vi "testUDPReciever - Copy 2.vi"() -> ()   [LabVIEW 2012]
panel:
  out "building array":string[](array[string])
  out "channel":u32
  out "header pre":bool[][](array[boolean])
  out "Found Header":bool
  out "word 0 pre":u8[](array[numeric]) format="%02x"
  out "word 1 pre":u8[](array[numeric]) format="%02x"
  out "word 2 pre":u8[](array[numeric]) format="%02x"
  out "word 3 pre":u8[](array[numeric]) format="%02x"
  out "Raw Data Out":string
  out "error post-check":errorcluster
  out "End Reciever Error":errorcluster
  in  "stop reciever":bool
  out "port":u16
  out "error out post-read":errorcluster
  out "error out pre-read":errorcluster
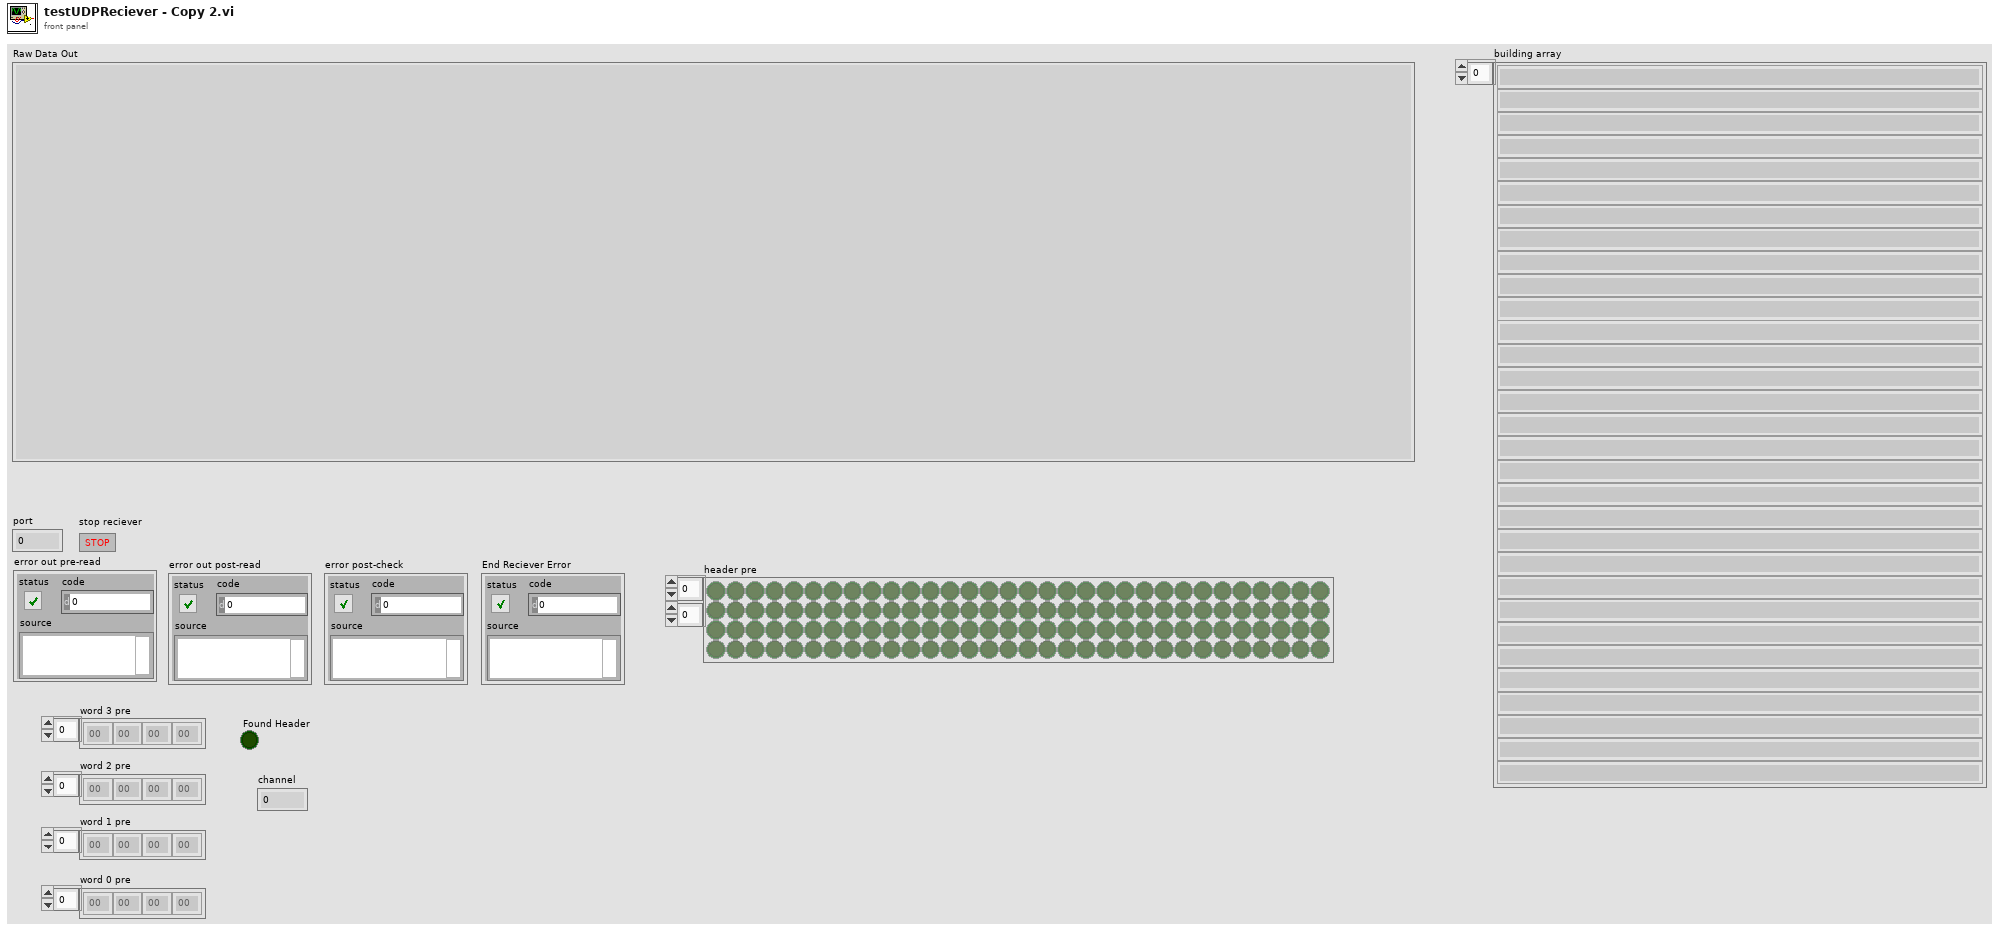
[diagram p1: front panel]
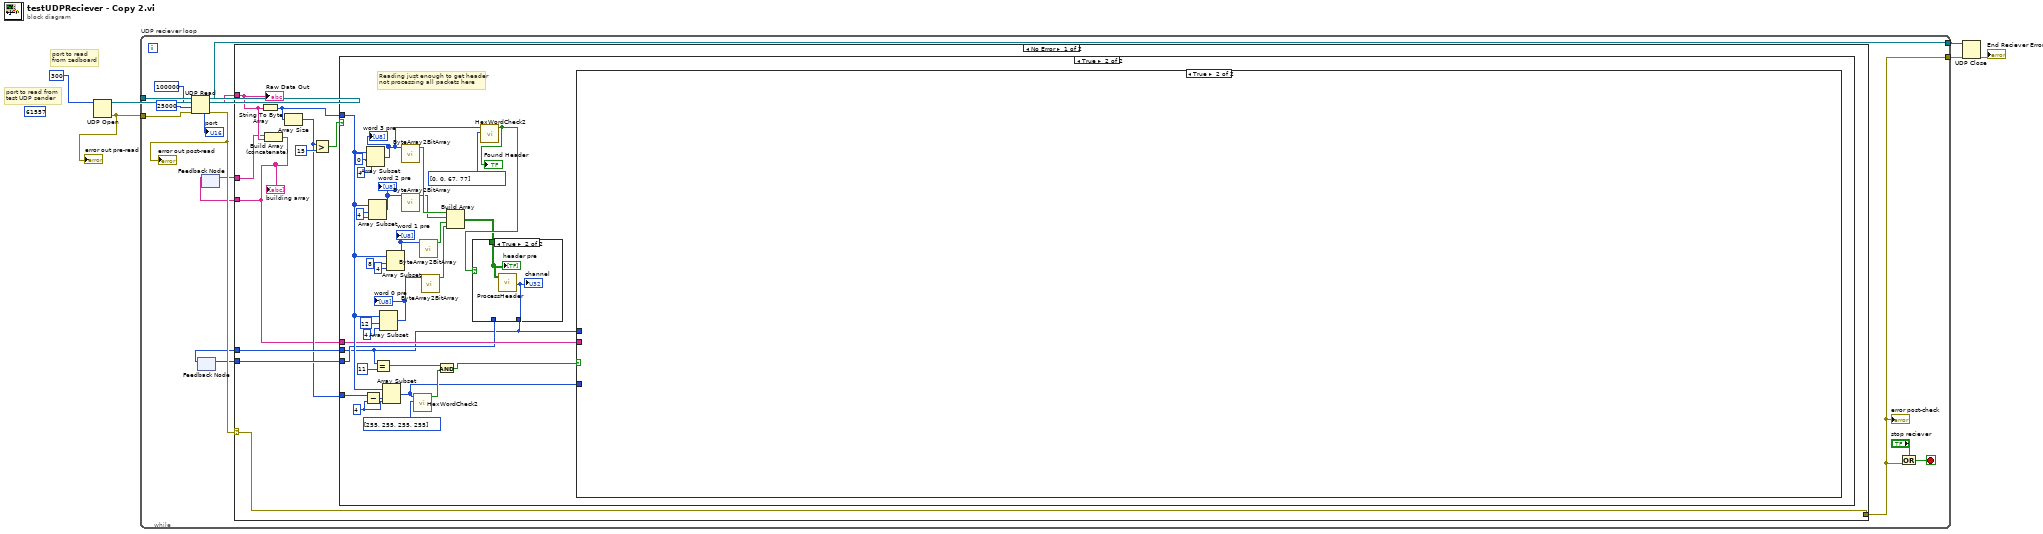
[diagram p0: block diagram]
diagram:
  (unwired) u16 61557 ("port")
  # "port to read \nfrom zedboard"
  # "port to read from \ntest UDP sender"
  n1 = UDP Open(11:u16 300 ("port")) -> (port=w5:refnum<k16>, 0:w2:errorcluster)  [unwired: 4 in, 1 out]
  "error out pre-read" <- w2
  n2 = while "UDP reciever loop" {
    tunnel: [w21] -> w6
    tunnel: w5 -> [w20]
    tunnel: [w12] -> w4
    tunnel: w2 -> [w17]
    stop <- w19 stop-if-true
    n3 = UDP Read(connection ID=w20, max size (548)=100000, timeout ms (25000)=25000, 8:w17) -> (data out=w14:string, error out=w16:errorcluster, 3:w21:refnum<k16>, 4:→"port":u16)  [unwired: 1 out]
    "error out post-read" <- w16
    n4 = feedback #1() -> (w7:u32)  [unwired: 1 in]
    n5 = feedback #2() -> (w9:string[])  [unwired: 1 in]
    n6 = case shown="No Error" w16 {
      selector: w16 -> [w31 w69]
      tunnel: w14 -> [w30 _]
      tunnel: [w31 w69] -> w12
      tunnel: [w23 w68] -> w10
      tunnel: w9 -> [w29 w68]
      tunnel: [w26 w67] -> w8
      tunnel: w7 -> [w25 w67]
      frame No Error {
        n7 = String To Byte Array(string=w30) -> (unsigned byte array=w22:u8[])
        n8 = Build Array (concatenate)(w29, w30) -> (w23:string[])
        "building array" <- w23
        n9 = Array Size(array=w22) -> (size(s)=w24:i32)
        n10 = Greater?(x=w24, y=15) -> (0:w28:bool)
        n11 = case shown="True" w28 {
          tunnel: w22 -> [_ w40]
          tunnel: [w32 w33] -> w26
          tunnel: w25 -> [w32 w34]
          tunnel: w24 -> [_ w37]
          tunnel: w23 -> [_ w36]
          frame False {
          }
          frame True {
            w39 = 4 ("length")
            w58 = 4 ("length")
            # "Reading just enough to get header\nnot processing all packets here"
            n12 = Subtract(x=w37, y=w39) -> (x-y=w38:i32)
            n13 = Array Subset(array=w40, index=0, length=4) -> (w47:u8[])
            "word 3 pre" <- w47
            n14 = Array Subset(array=w40, index=w58, length=w58) -> (w63:u8[])
            "word 2 pre" <- w63
            n15 = Array Subset(array=w40, index=12, length=4) -> (w45:u8[])
            "word 0 pre" <- w45
            n16 = Array Subset(array=w40, index=w38, length=w39) -> (w35:u8[])
            n17 = Array Subset(array=w40, index=8, length=4) -> (w62:u8[])
            "word 1 pre" <- w62
            n18 = call "ByteArray2BitArray.vi"("array"=w47) -> ("Array"=w53:bool[])  [unwired: 10 in]
            n19 = call "ByteArray2BitArray.vi"("array"=w63) -> ("Array"=w52:bool[])  [unwired: 10 in]
            n20 = call "HexWordCheck2.vi"("array"=u8[] [255, 255, 255, 255], "Input Array"=w35) -> ("Boolean"=w41:bool)  [unwired: 9 in]
            n21 = call "ByteArray2BitArray.vi"("array"=w62) -> ("Array"=w50:bool[])  [unwired: 10 in]
            n22 = call "ByteArray2BitArray.vi"("array"=w45) -> ("Array"=w51:bool[])  [unwired: 10 in]
            n23 = Build Array(w53, w52, w50, w51) -> (w48:bool[][])
            n24 = call "HexWordCheck2.vi"("array"=u8[] [0, 0, 67, 77], "Input Array"=w47) -> ("Boolean"=w49:bool)  [unwired: 9 in]
            "Found Header" <- w49
            n25 = case shown="True" w49 {
              tunnel: w48 -> [_ w66]
              tunnel: [w64 w65] -> w33
              tunnel: w34 -> [w64 _]
              frame False {
              }
              frame True {
                n26 = call "ProcessHeader.vi"("Array"=w66) -> ("Numeric 4"=w65:u32)  [unwired: 4 in, 6 out]
                "channel" <- w65
                "header pre" <- w66
              }
            }
            n27 = Equal?(x=w33, y=u32 11) -> (x = y?=w42:bool)
            n28 = And(x=w42, y=w41) -> (x .and. y?=w44:bool)
            n29 = case shown="True" w44 {
              tunnel: w36 -> [_ _]
              tunnel: w33 -> [_ _]
              tunnel: w35 -> [_ _]
              frame False {
              }
              frame True {
              }
            }
          }
        }
        "Raw Data Out" <- w30
      }
      frame Error {
      }
    }
    "error post-check" <- w12
    n30 = feedback-in #1(w8) -> ()
    n31 = feedback-in #2(w10) -> ()
    n32 = Or(x="stop reciever", y=w12) -> (x .or. y?=w19:bool)
  }
  n33 = UDP Close(connection ID=w6, 8:w4) -> (error out=→"End Reciever Error":errorcluster)  [unwired: 1 out]
